vi "Get Item Display Name.vi"(8 "error in (no error)":errorcluster, 9 "Tag":string, 11 "TreeControl in":refnum<vi>) -> (0 "error out":errorcluster, 2 "display name":string, 3 "TreeControl out":refnum<vi>)   [LabVIEW 2017, in "DSF Simple Explorer.lvlib"]
uses:
  DSF Simple Explorer.lvlib
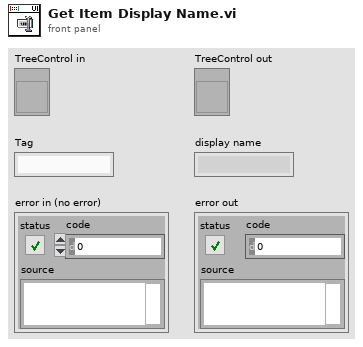
[diagram p1: front panel]
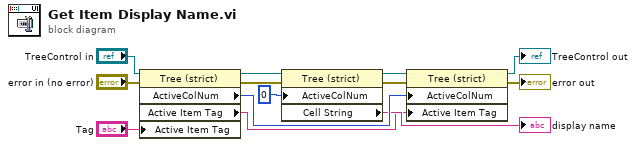
[diagram p0: block diagram]
diagram:
  n1 = property class="Tree (strict)"(reference="TreeControl in", error in="error in (no error)", "Active Item Tag"="Tag") -> (reference out=w5:refnum<vi>, error out=w8:errorcluster, "ActiveColNum"=w7:i32, "Active Item Tag"=w1:string)
  n2 = property class="Tree (strict)"(reference=w5, error in=w8, "ActiveColNum"=0 ("Active Cell:Active Column Number")) -> (reference out=w6:refnum<vi>, error out=w9:errorcluster, "Cell String"=→"display name":string)
  n3 = property class="Tree (strict)"(reference=w6, error in=w9, "ActiveColNum"=w7, "Active Item Tag"=w1) -> (reference out=→"TreeControl out":refnum<vi>, error out=→"error out":errorcluster)
